vi "Query Marker.vi"(8 "error in (no error)":errorcluster, 10 "Marker Number (1)":u32=1 min=1, 11 "SA-FSW in":refnum<class "SA-FSW.lvclass">) -> (0 "error out":errorcluster, 1 "Marker Level":dbl, 2 "Marker Frequency/Time":dbl, 3 "SA-FSW out":refnum<class "SA-FSW.lvclass">)   [LabVIEW 2020, in "SA-FSW.lvclass"]
uses:
  SA-FSW.lvclass
  C:/Sandbox/Git_Sandbox/WiSpry Test Framework source code (LV20)/WiSpry Test Framework/Instruments/Instrument.lvclass
  Instrument.lvclass/Instrument.ctl
  Instrument.lvclass
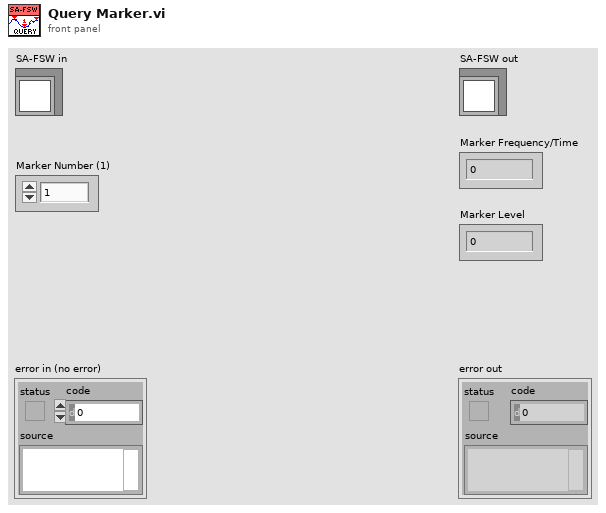
[diagram p1: front panel]
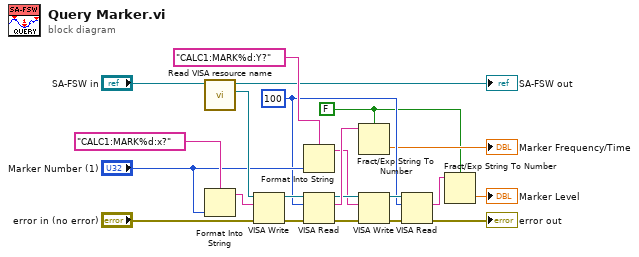
[diagram p0: block diagram]
diagram:
  w7 = u32 100 ("byte count")
  w3 = FALSE ("use system decimal point (T)")
  n1 = call "Read VISA resource name.vi"("Instrument in"="SA-FSW in") -> ("VISA resource name"=w20:refnum<visa-resource-name>, "Instrument out"=→"SA-FSW out":refnum<class "SA-FSW.lvclass">)  [unwired: 9 in]
  n2 = Format Into String(format string="CALC1:MARK%d:x?", "Marker Number (1)") -> (resulting string=w19:string)  [unwired: 2 in, 1 out]
  n3 = VISA Write(VISA resource name=w20, write buffer=w19, error in (no error)="error in (no error)") -> (VISA resource name out=w16:refnum<visa-resource-name>, error out=w17:errorcluster)  [unwired: 1 out]
  n4 = Format Into String(format string="CALC1:MARK%d:Y?", "Marker Number (1)") -> (resulting string=w10:string)  [unwired: 2 in, 1 out]
  n5 = VISA Read(VISA resource name=w16, byte count=w7, error in (no error)=w17) -> (VISA resource name out=w11:refnum<visa-resource-name>, read buffer=w15:string, error out=w12:errorcluster)  [unwired: 1 out]
  n6 = Fract/Exp String To Number(use system decimal point (T)=w3, string=w15) -> (number=→"Marker Frequency/Time":dbl)  [unwired: 2 in, 1 out]
  n7 = VISA Write(VISA resource name=w11, write buffer=w10, error in (no error)=w12) -> (VISA resource name out=w8:refnum<visa-resource-name>, error out=w9:errorcluster)  [unwired: 1 out]
  n8 = VISA Read(VISA resource name=w8, byte count=w7, error in (no error)=w9) -> (read buffer=w5:string, error out=→"error out":errorcluster)  [unwired: 2 out]
  n9 = Fract/Exp String To Number(use system decimal point (T)=w3, string=w5) -> (number=→"Marker Level":dbl)  [unwired: 2 in, 1 out]
